vi "Diagrama final con subvi.vi"() -> ()   [LabVIEW 2022 SP3]
uses:
  <vilib>/Instr/_visa.llb/VISA Configure Serial Port (Instr).vi
panel:
  out "MODO OPERACION":bool
  in  "ENVIAR_CONFI":bool
  in  "ALTO":bool
  in  "Configuracion ADS1263":T1 {"Muestras" items=["50", "250", "1000", "2000", "5000", "10000", "15000", "30000"]; "PGA" items=["1", "2", "4", "8", "16", "32"]; "Muestreo" items=["2.5 SPS", "5 SPS", "10 SPS", "16.6 SPS", "20 SPS", "50 SPS", "60 SPS", "100 SPS", "400 SPS", "1200 SPS", "2400 SPS", "4800 SPS", "7200 SPS", "14400 SPS", "19200 SPS", "38400 SPS"]}
  out "s? t:f":u8
  in  "Inicializacion LoRa":T2={"Enviar direccion"=FALSE, "Direccion"=1} {"Direccion" min=1 max=127 step=1}
  in  "VISA resource name":refnum<visa-resource-name>
  in  "ABORTAR":bool
  # "Velocidad de muestreo"
  # "PGA del sistema"
  # "HABILITAR MODO DIFERENCIAL 1 Y 2"
  # "HABILITAR MODO DIFERENCIAL 3 Y 4"
  # "FILTRO PARA AC1 Y AC2"
  # "100Hz"
  # "500Hz"
  # "FILTRO PARA AC3 Y AC4"
  # "100Hz"
  # "500Hz"
  # "MODO DE OPERACION DEMANDA"
  # "MODO DE OPERACION CONTROLADA"
  # "Cantidad de muestras tomadas"
  # "Recibir por LoRa"
  # "Recibir por SD"
  # "Direccion fisiografo (1-127)"
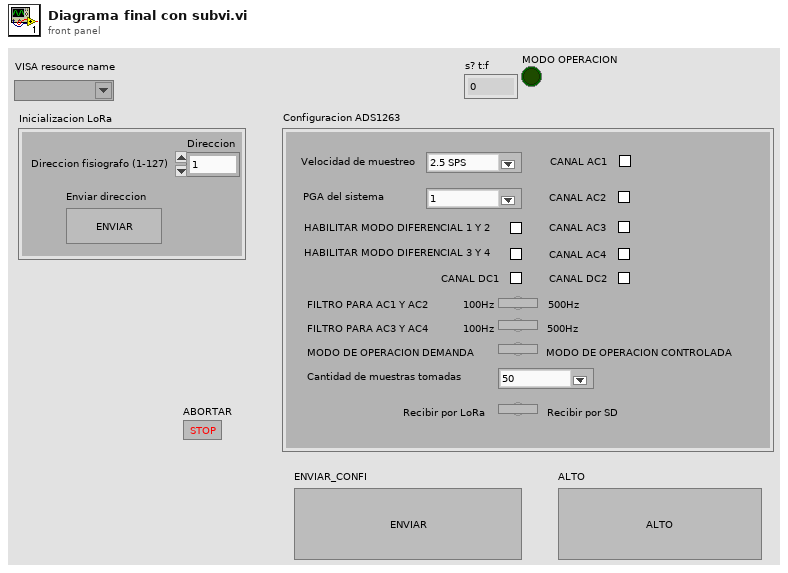
[diagram p1: front panel]
types:
  T1 = cluster{"Muestreo":u32, "PGA":u32, "DIF1Y2":bool, "DIF3Y4":bool, "CANAL AC1":bool, "CANAL AC2":bool, "CANAL AC3":bool, "CANAL AC4":bool, "CANAL DC1":bool, "CANAL DC2":bool, "FILTRO1":bool, "FILTRO2":bool, "MODO OPERACION":bool, "Muestras":u32, "MODO transmision":bool}
  T2 = cluster{"Enviar direccion":bool, "Direccion":i16}
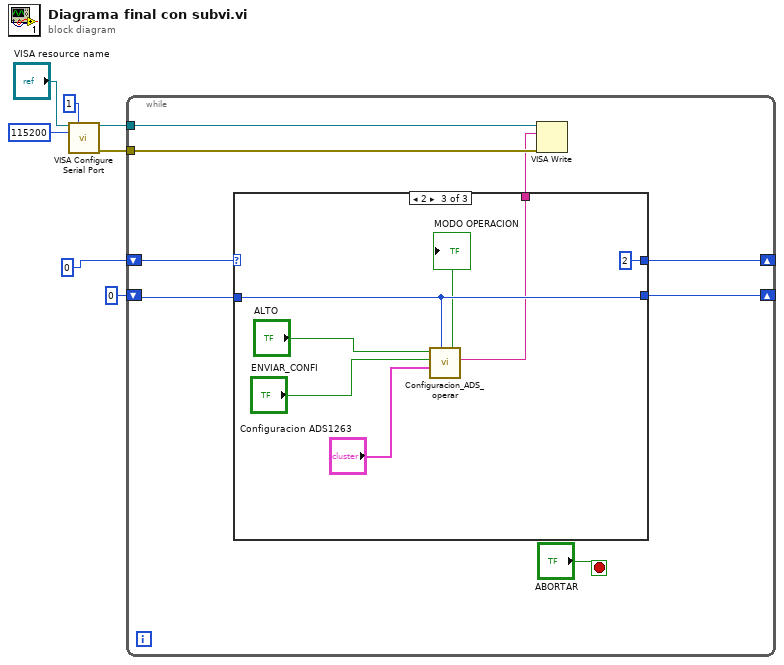
[diagram p0: block diagram]
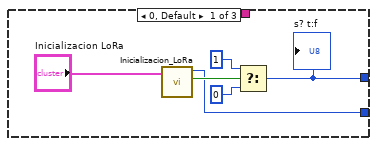
[diagram p2: hidden frame]
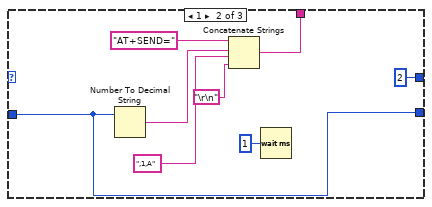
[diagram p3: hidden frame]
diagram:
  n1 = call-poly "VISA Configure Serial Port"("VISA resource name"="VISA resource name", "timeout (10sec)"=u32 1, "baud rate (9600)"=u32 115200) -> ("VISA resource name out"=w7:refnum<visa-resource-name>, "error out"=w3:errorcluster)  [unwired: 11 in]
  n2 = while {
    tunnel: w7 -> [w10]
    tunnel: w3 -> [w9]
    shift-right: [w13] -> _
    shift-left: u8 0 ("baud rate (9600)") -> [w14]
    shift-right: [w12] -> _
    shift-left: i16 0 ("Direccion") -> [w11]
    stop <- "ABORTAR" stop-if-true
    n3 = case shown="2" w14 {
      tunnel: [w19 u8 2 ("f") u8 2 ("f")] -> w13
      tunnel: [w16 w22 w35] -> w12
      tunnel: w11 -> [_ w22 w35]
      tunnel: [_ w25 w30] -> w8
      frame 0, Default {
        n4 = call "Inicializacion_LoRa.vi"("Inicializacion LoRa"="Inicializacion LoRa") -> ("Enviar direccion"=w20:bool, "Direccion"=w16:i16)  [unwired: 9 in]
        n5 = Select(t=u8 1, s=w20, f=u8 0) -> (s? t:f=w19:u8)
        "s? t:f" <- w19
      }
      frame 1 {
        n6 = Number To Decimal String(number=w22) -> (decimal integer string=w28:string)  [unwired: 1 in]
        n7 = Concatenate Strings("AT+SEND=" ("string"), w28, ",1,A" ("string"), "\r\n") -> (w25:string)
        n8 = Wait (ms)(milliseconds to wait=u32 1) -> ()  [unwired: 1 out]
      }
      frame 2 {
        n9 = call "Configuracion_ADS_operar.vi"("Direccion"=w35, "Configuracion ADS1263"="Configuracion ADS1263", "ENVIAR_CONFI"="ENVIAR_CONFI", "ALTO"="ALTO") -> ("concatenated string"=w30:string, "MODO OPERACION"=→"MODO OPERACION":bool)  [unwired: 6 in]
      }
    }
    n10 = VISA Write(VISA resource name=w10, write buffer=w8, error in (no error)=w9) -> ()  [unwired: 3 out]
  }
